vi "create.vi"(8 "error in (no error)":errorcluster, 9 "maximum":refnum<class "SpaceVector.lvclass">, 10 "minimum":refnum<class "SpaceVector.lvclass">) -> (0 "error out":errorcluster, 3 "Box out":refnum<class "Box.lvclass">)   [LabVIEW 2010, in "Box.lvclass"]
uses:
  Box.lvclass
  SpaceVector/SpaceVector/SpaceVector.lvclass
  Box.lvclass/Box.ctl
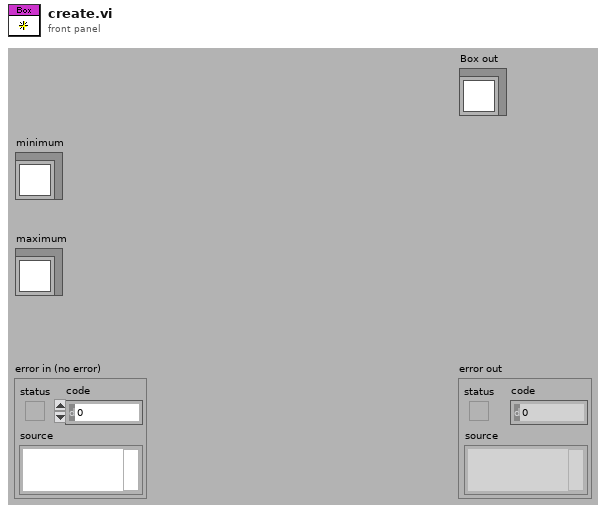
[diagram p1: front panel]
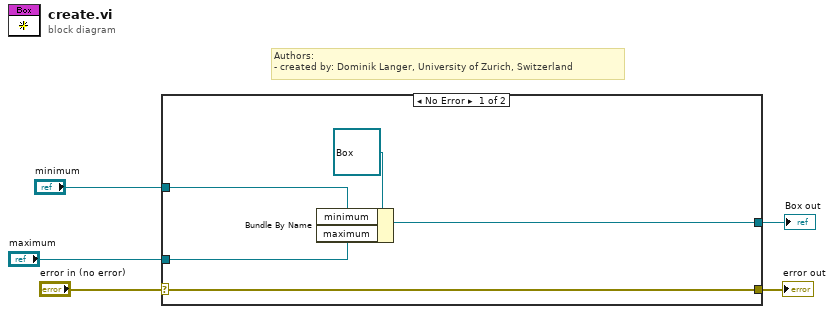
[diagram p0: block diagram]
diagram:
  # "Authors: \n- created by: Dominik Langer, University of Zurich, Switzerland"
  n1 = case shown="No Error" "error in (no error)" {
    selector: "error in (no error)" -> [w10 w11]
    tunnel: [w10 w11] -> w4
    tunnel: [w9 _] -> w3
    tunnel: "minimum" -> [w8 _]
    tunnel: "maximum" -> [w7 _]
    frame No Error {
      n2 = Bundle By Name(cluster=refnum<class "Box.lvclass"> refnum ("Box.lvclass"), "minimum"=w8, "maximum"=w7) -> (w9:refnum<class "Box.lvclass">)
    }
    frame Error {
    }
  }
  "error out" <- w4
  "Box out" <- w3
